vi "RTMain.Refs.Initialize.vi"(8 "error in (no error)":errorcluster, 11 "VS References":T1={"Name"="", "CAN"={"Interface"="", "Baud Rate"=0, "Diagnostic Protocol"=enum."GMLAN", "Transport Protocol"=enum."ISO TP - Normal Mode", "Transmit ID"=0, "Receive ID"=2, "Transmit Extension"=1, "Receive Extension"=255, "Receive UUDT ID"=0, "Enable Stream"=TRUE, "VW TP Channel ID"=1, "Fill Frame"=FALSE, "Fill Byte"=0, "Termination"=FALSE, "LIN Cluster"="", "NAD"=8, "IO Mode"=0, "Max DLC"=0, "FD Baud Rate"=2, "Timeout"=1}, "986x"={"Enable"=FALSE, "RIO Device"="", "Bitfile"=path ""}, "Reads"=[], "Frames Lookup"=variant(enum16{"GMLAN", "KWP-2000", "UDS"} enum."GMLAN"), "Writes"=[], "DPIDs"=[], "DPID Lookup"=variant(u32 0), "DTC"={"Descriptor"={"DTC Byte Length"=1, "Status Byte Length"=1, "Add Data Byte Length"=1, "Byte Order"=enum."Motorola"}, "Value.Code"=[], "Value.String"=[], "Value.J2012String"=[], "Status.Code"=[], "Status.String"=[]}, "Created DTCs"=0, "Polls"=[], "Service Channels Status Lookup"=variant, "Trigger Lookup"=variant, "Security"={"Type"=enum."None", "Source DLL Path"=path "", "Target DLL Path"=path "", "Security Level"=0}} {"Writes"."Signals"."Byte Order" items=["Little Endian", "Big Endian"]; "Writes"."Signals"."Data Type" items=["Signed", "Unsigned", "IEEE Float"]; "CAN"."IO Mode" items=["CAN 2.0", "CAN FD", "CAN FD+BRS"]; "CAN"."Fill Byte" format="%.0x"; "CAN"."VW TP Channel ID" format="%.0x"; "CAN"."Receive UUDT ID" format="%.0x"; "CAN"."Receive Extension" format="%.0x"; "CAN"."Transmit Extension" format="%.0x"; "CAN"."Receive ID" format="%.0x"; "CAN"."Transmit ID" format="%.0x"; "Reads"."Signals"."Byte Order" items=["Little Endian", "Big Endian"]; "Reads"."Signals"."Data Type" items=["Signed", "Unsigned", "IEEE Float"]}) -> (0 "error out":errorcluster, 2 "FPGA Session":u32, 3 "VS Main Configuration":T1={"Name"="", "CAN"={"Interface"="", "Baud Rate"=0, "Diagnostic Protocol"=enum."GMLAN", "Transport Protocol"=enum."ISO TP - Normal Mode", "Transmit ID"=0, "Receive ID"=2, "Transmit Extension"=1, "Receive Extension"=255, "Receive UUDT ID"=0, "Enable Stream"=TRUE, "VW TP Channel ID"=1, "Fill Frame"=FALSE, "Fill Byte"=0, "Termination"=FALSE, "LIN Cluster"="", "NAD"=8, "IO Mode"=0, "Max DLC"=0, "FD Baud Rate"=2, "Timeout"=1}, "986x"={"Enable"=FALSE, "RIO Device"="", "Bitfile"=path ""}, "Reads"=[], "Frames Lookup"=variant(enum16{"GMLAN", "KWP-2000", "UDS"} enum."GMLAN"), "Writes"=[], "DPIDs"=[], "DPID Lookup"=variant(u32 0), "DTC"={"Descriptor"={"DTC Byte Length"=1, "Status Byte Length"=1, "Add Data Byte Length"=1, "Byte Order"=enum."Motorola"}, "Value.Code"=[], "Value.String"=[], "Value.J2012String"=[], "Status.Code"=[], "Status.String"=[]}, "Created DTCs"=0, "Polls"=[], "Service Channels Status Lookup"=variant, "Trigger Lookup"=variant, "Security"={"Type"=enum."None", "Source DLL Path"=path "", "Target DLL Path"=path "", "Security Level"=0}} {"Writes"."Signals"."Byte Order" items=["Little Endian", "Big Endian"]; "Writes"."Signals"."Data Type" items=["Signed", "Unsigned", "IEEE Float"]; "CAN"."IO Mode" items=["CAN 2.0", "CAN FD", "CAN FD+BRS"]; "CAN"."Fill Byte" format="%.0x"; "CAN"."VW TP Channel ID" format="%.0x"; "CAN"."Receive UUDT ID" format="%.0x"; "CAN"."Receive Extension" format="%.0x"; "CAN"."Transmit Extension" format="%.0x"; "CAN"."Receive ID" format="%.0x"; "CAN"."Transmit ID" format="%.0x"; "Reads"."Signals"."Byte Order" items=["Little Endian", "Big Endian"]; "Reads"."Signals"."Data Type" items=["Signed", "Unsigned", "IEEE Float"]})   [LabVIEW 2019, in "Diagnostics Addon Engine.lvlib"]
uses:
  Diagnostics Addon Engine.lvlib
  Addon Shared/Types/SysDef.Compile.ctl
  Addon Shared/Types/CAN.ctl
  Addon Shared/Types/CAN.Interface.ctl
  Addon Shared/Types/Protocol.ctl
  Addon Shared/Types/Transport.ctl
  Addon Shared/Types/986x.ctl
  Addon Shared/Types/Frame.Compile.ctl
  Addon Shared/Types/Type.ctl
  Addon Shared/Types/Signal.ctl
  Addon Shared/Types/DPID.ctl
  Addon Shared/Types/DPID.Rate.ctl
  Addon Shared/Types/DTC.Settings.ctl
  Addon Shared/Types/DTC.Descriptor.ctl
  Addon Shared/Types/Poll.Compiled.ctl
  Addon Shared/Types/Security.ctl
  Addon Shared/Types/Security.Type.ctl
  Addon Shared/Diagnostics Addon Shared.lvlib
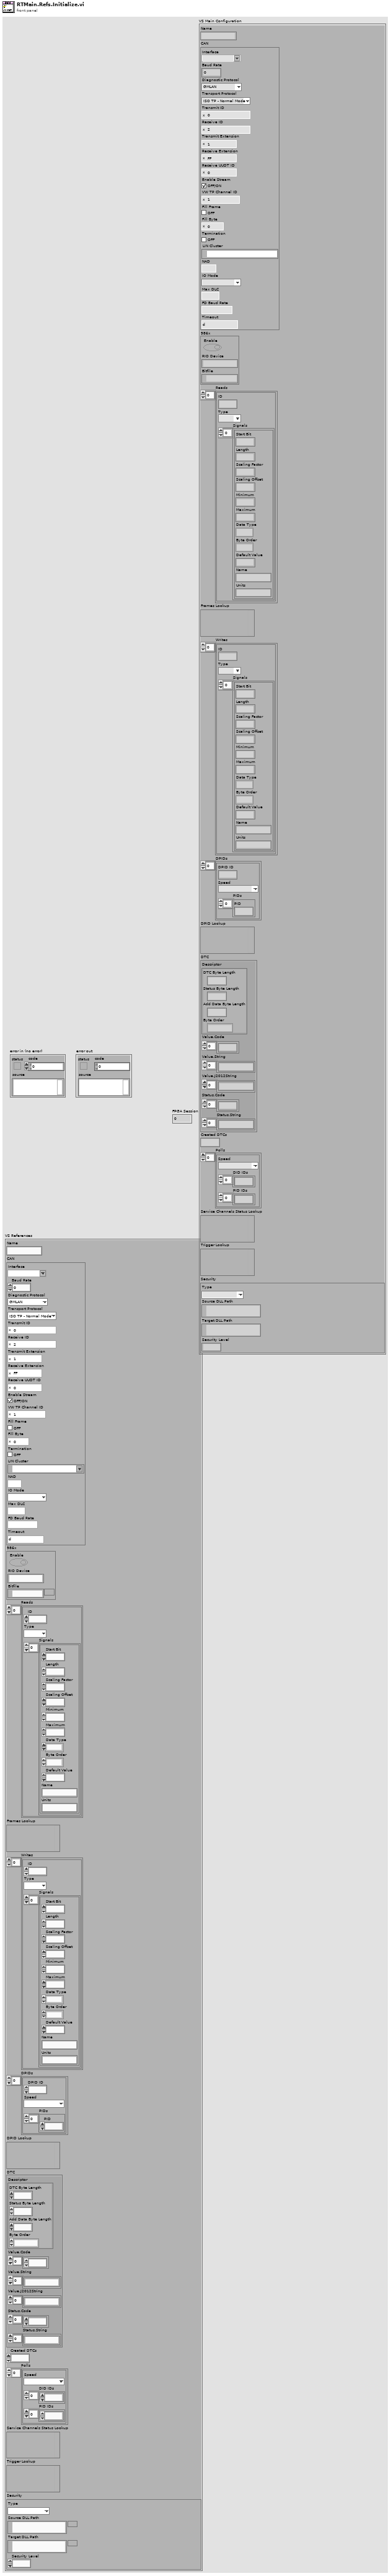
[diagram p1: front panel]
types:
  T1 = typedef "Diagnostics Addon Shared.lvlib/SysDef.Compile.ctl" = cluster{"Name":string, "CAN":T2, "986x":T6, "Reads":T7[], "Frames Lookup":variant, "Writes":T7[], "DPIDs":T10[], "DPID Lookup":variant, "DTC":T12, "Created DTCs":u32, "Polls":T14[], "Service Channels Status Lookup":variant, "Trigger Lookup":variant, "Security":T15}
  T2 = typedef "Diagnostics Addon Shared.lvlib/CAN.ctl" = cluster{"Interface":T3, "Baud Rate":u64, "Diagnostic Protocol":T4, "Transport Protocol":T5, "Transmit ID":u32, "Receive ID":u32, "Transmit Extension":u8, "Receive Extension":u8, "Receive UUDT ID":u32, "Enable Stream":bool, "VW TP Channel ID":u32, "Fill Frame":bool, "Fill Byte":u8, "Termination":bool, "LIN Cluster":refnum<k21>, "NAD":u8, "IO Mode":u32, "Max DLC":u16, "FD Baud Rate":u64, "Timeout":u32}
  T3 = typedef "Diagnostics Addon Shared.lvlib/CAN.Interface.ctl" = string
  T4 = typedef "Diagnostics Addon Shared.lvlib/Protocol.ctl" = enum16{"GMLAN", "KWP-2000", "UDS", "User-Defined"}
  T5 = typedef "Diagnostics Addon Shared.lvlib/Transport.ctl" = enum16{"ISO TP - Normal Mode", "ISO TP - Mixed Mode", "VW TP 2.0", "Diagnostics on IP", "ISO TP LIN"}
  T6 = typedef "Diagnostics Addon Shared.lvlib/986x.ctl" = cluster{"Enable":bool, "RIO Device":string, "Bitfile":path}
  T7 = typedef "Diagnostics Addon Shared.lvlib/Frame.Compile.ctl" = cluster{"ID":u32, "Type":T8, "Signals":T9[]}
  T8 = typedef "Diagnostics Addon Shared.lvlib/Type.ctl" = enum16{"DID", "CDID", "PID", "CPID", "Read Memory", "Write Memory", "IO Control", "Routine Start", "Routine Request", "Routine Stop", "User Defined", "DTC Control", "Clear DTCs", "Read DTCs", "Start DTCs", "DTC Change Count", "Tester Present", "Unlock ECU", "Reset ECU", "Diag Session Control", "Communication Control", "DPID Control", "Poll Control", "Diag CAN Control"}
  T9 = typedef "Diagnostics Addon Shared.lvlib/Signal.ctl" = cluster{"Start Bit":u32, "Length":u32, "Scaling Factor":dbl, "Scaling Offset":dbl, "Minimum":dbl, "Maximum":dbl, "Data Type":u32, "Byte Order":u32, "Default Value":dbl, "Name":string, "Units":string}
  T10 = typedef "Diagnostics Addon Shared.lvlib/DPID.ctl" = cluster{"DPID ID":u8, "Speed":T11, "PIDs":u16[]}
  T11 = typedef "Diagnostics Addon Shared.lvlib/DPID.Rate.ctl" = enum16{"Slow", "Medium", "Fast"}
  T12 = typedef "Diagnostics Addon Shared.lvlib/DTC.Settings.ctl" = cluster{"Descriptor":T13, "Value.Code":dbl[], "Value.String":string[], "Value.J2012String":string[], "Status.Code":dbl[], "Status.String":string[]}
  T13 = typedef "Diagnostics Addon Shared.lvlib/DTC.Descriptor.ctl" = cluster{"DTC Byte Length":i32, "Status Byte Length":i32, "Add Data Byte Length":i32, "Byte Order":enum16{"Motorola", "Intel"}}
  T14 = typedef "Diagnostics Addon Shared.lvlib/Poll.Compiled.ctl" = cluster{"Speed":T11, "DID IDs":u32[], "PID IDs":u32[]}
  T15 = typedef "Diagnostics Addon Shared.lvlib/Security.ctl" = cluster{"Type":T16, "Source DLL Path":path, "Target DLL Path":path, "Security Level":u8}
  T16 = typedef "Diagnostics Addon Shared.lvlib/Security.Type.ctl" = enum16{"None", "DLL", "MasterKey"}
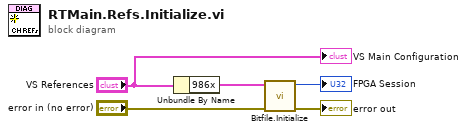
[diagram p0: block diagram]
diagram:
  n1 = Unbundle By Name("VS References") -> ("986x"=w3:T6)
  n2 = call "Bitfile.Initialize.vi"("error in (no error)"="error in (no error)", "FPGA Bitfile Settings"=w3) -> ("error out"=→"error out":errorcluster, "FPGA Session"=→"FPGA Session":u32)  [unwired: 8 in]
  "VS Main Configuration" <- "VS References"
